vi "Set Process Qs.vi"(10 "Process Qs":refnum<queue>[](array[refnum]), 11 "Process in":refnum<class "Process.lvclass">) -> (3 "Process out":refnum<class "Process.lvclass">)   [LabVIEW 2019, in "TimingDRV Engine.lvlib" / "Process.lvclass"]
uses:
  Process.lvclass
  TypeDefs/Message.ctl
  Process.lvclass/Process.ctl
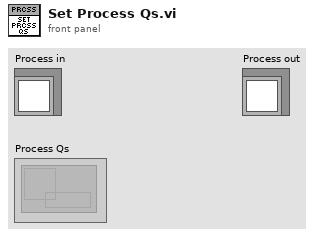
[diagram p1: front panel]
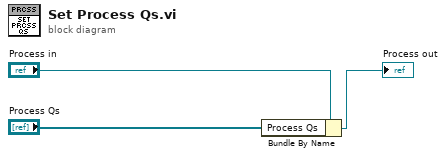
[diagram p0: block diagram]
diagram:
  n1 = Bundle By Name(cluster="Process in", "Process Qs"="Process Qs") -> (→"Process out":refnum<class "Process.lvclass">)
